vi "Find Sheet Bounds.vi"(8 "error in (no error)":errorcluster, 11 "Excel in":refnum<class "Excel.lvclass">) -> (0 "error out":errorcluster, 2 "Bounding Cell":cluster{"Row":i32, "Column":i32}, 3 "Excel out":refnum<class "Excel.lvclass">, 4 "Bounding Column ++":cluster{"Row":i32, "Column":i32}, 5 "Bounding Column":cluster{"Row":i32, "Column":i32}, 6 "Bounding Row ++":cluster{"Row":i32, "Column":i32}, 7 "Bounding Row":cluster{"Row":i32, "Column":i32})   [LabVIEW 2016, in "Excel.lvclass"]
uses:
  Excel.lvclass
  Excel.lvclass/Excel.ctl
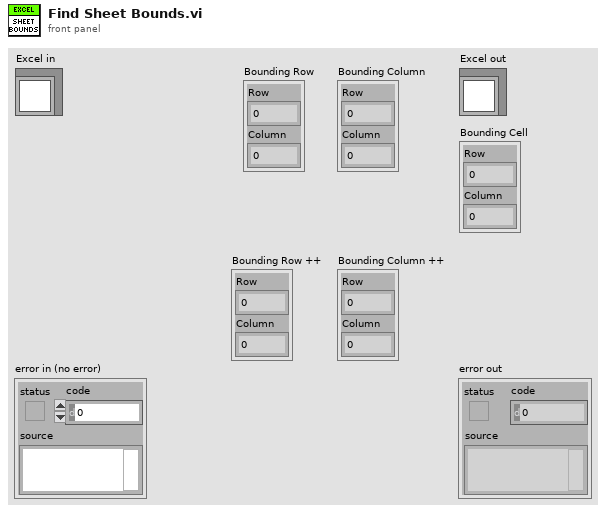
[diagram p1: front panel]
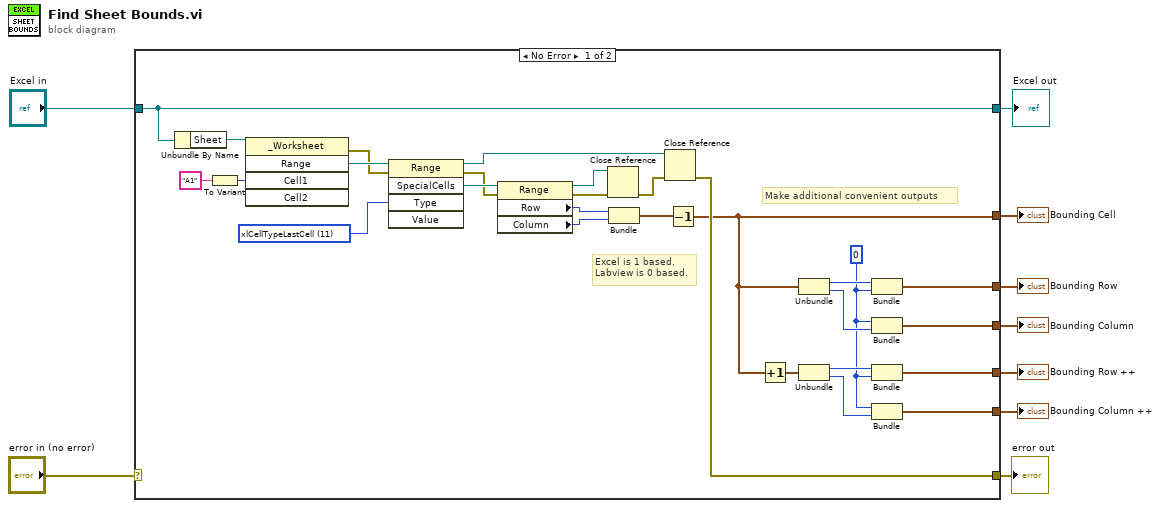
[diagram p0: block diagram]
diagram:
  n1 = case shown="No Error" "error in (no error)" {
    selector: "error in (no error)" -> [_ w39]
    tunnel: [w24 w39] -> w8
    tunnel: [w37 w38] -> w6
    tunnel: "Excel in" -> [w37 w38]
    tunnel: [w18 _] -> w5
    tunnel: [w13 _] -> w4
    tunnel: [w12 _] -> w3
    tunnel: [w11 _] -> w2
    tunnel: [w10 _] -> w1
    frame No Error {
      w15 = 0
      w32 = 11 items=["xlCellTypeBlanks"=4, "xlCellTypeConstants"=2, "xlCellTypeFormulas"=-4123, "xlCellTypeLastCell"=11, "xlCellTypeComments"=-4144, "xlCellTypeVisible"=12, "xlCellTypeAllFormatConditions"=-4172, "xlCellTypeSameFormatConditions"=-4173, "xlCellTypeAllValidation"=-4174, "xlCellTypeSameValidation"=-4175] ("Type")
      # "Make additional convenient outputs"
      # "Excel is 1 based.\nLabview is 0 based."
      n2 = Unbundle By Name(w37) -> ("Sheet"=w36:refnum<k7>)
      n3 = To Variant(anything="A1") -> (Variant=w34:variant)
      n4 = invoke class="_Worksheet" method="Range"(reference=w36, "Cell1"=w34) -> (error out=w29:errorcluster, "Range"=w33:refnum<k7>)  [unwired: 3 in, 3 out]
      n5 = invoke class="Range" method="SpecialCells"(reference=w33, error in=w29, "Type"=w32) -> (reference out=w26:refnum<k7>, error out=w30:errorcluster, "SpecialCells"=w31:refnum<k7>)  [unwired: 2 in, 2 out]
      n6 = property class="Range"(reference=w31, error in=w30) -> (reference out=w28:refnum<k7>, error out=w27:errorcluster, "Row"=w23:i32, "Column"=w22:i32)
      n7 = Close Reference(reference=w28, error in (no error)=w27) -> (error out=w25:errorcluster)
      n8 = Bundle("Row"=w23, "Column"=w22) -> (w21:cluster{"Row":i32, "Column":i32})  [unwired: 1 in]
      n9 = Close Reference(reference=w26, error in (no error)=w25) -> (error out=w24:errorcluster)
      n10 = Decrement(x=w21) -> (x-1=w18:cluster{"Row":i32, "Column":i32})
      n11 = Increment(x=w18) -> (x+1=w14:cluster{"Row":i32, "Column":i32})
      n12 = Unbundle(w18) -> ("Row"=w20:i32, "Column"=w19:i32)
      n13 = Unbundle(w14) -> ("Row"=w16:i32, "Column"=w17:i32)
      n14 = Bundle("Row"=w20, w15) -> (w13:cluster{"Row":i32, i32})  [unwired: 1 in]
      n15 = Bundle(w15, "Column"=w19) -> (w12:cluster{i32, "Column":i32})  [unwired: 1 in]
      n16 = Bundle("Row"=w16, w15) -> (w11:cluster{"Row":i32, i32})  [unwired: 1 in]
      n17 = Bundle(w15, "Column"=w17) -> (w10:cluster{i32, "Column":i32})  [unwired: 1 in]
    }
    frame Error {
    }
  }
  "error out" <- w8
  "Excel out" <- w6
  "Bounding Cell" <- w5
  "Bounding Row" <- w4
  "Bounding Column" <- w3
  "Bounding Row ++" <- w2
  "Bounding Column ++" <- w1
